vi "DSF.Shared.Configuration.Set Name.vi"(10 "Name":string, 11 "Configuration in":refnum<class "DSF.Shared.Configuration.lvclass">) -> (3 "Configuration out":refnum<class "DSF.Shared.Configuration.lvclass">)   [LabVIEW 2016, in "DSF.Shared.lvlib" / "DSF.Shared.Configuration.lvclass"]
uses:
  DSF.Shared.Configuration.lvclass
  DSF.Shared.Configuration.lvclass/DSF.Shared.Configuration.ctl
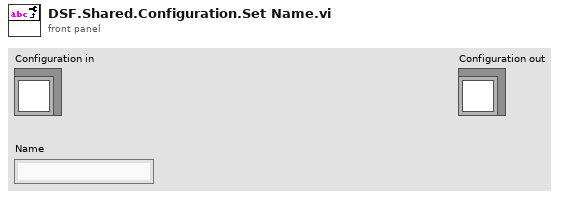
[diagram p1: front panel]
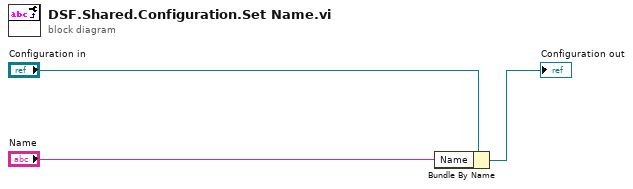
[diagram p0: block diagram]
diagram:
  n1 = Bundle By Name(cluster="Configuration in", "Name"="Name") -> (→"Configuration out":refnum<class "DSF.Shared.Configuration.lvclass">)
